vi "CODMn通讯.vi"() -> ()   [LabVIEW 2016, in "斯坦道CODMn.lvlib"]
uses:
  <vilib>/NI/Modbus Library/API/Wrapper/Create TCP Slave.vi
  <vilib>/NI/Modbus Library/API/slave/Modbus Slave.lvclass
  <vilib>/Plasmionique/MB Master/MB_Master/MB_Master.lvclass
  <vilib>/Plasmionique/MB Master/MB Master.lvlib
  <vilib>/Utility/config.llb/NI_LVConfig.lvlib
  <vilib>/NI/Modbus Library/API/Wrapper/API Main.lvlib
panel:
  in  "读取数据":bool
  in  "释放串口":bool
  in  "打开串口":bool
  out "队列中元素数量":i32
  out "元素":cluster{"命令":string}[](array[cluster])
  out "待处理插入数量":i32
  out "读取公式":u16[](array[numeric])
  out "读取参数":u16[](array[numeric])
  out "数据存储":u16[](array[numeric])
  out "温度":bool[](array[boolean])
  out "M输出点":bool[](array[boolean])
  out "ORP、时间":u16[](array[numeric])
  out "测量状态":u16[](array[numeric])
  out "通讯状态":bool
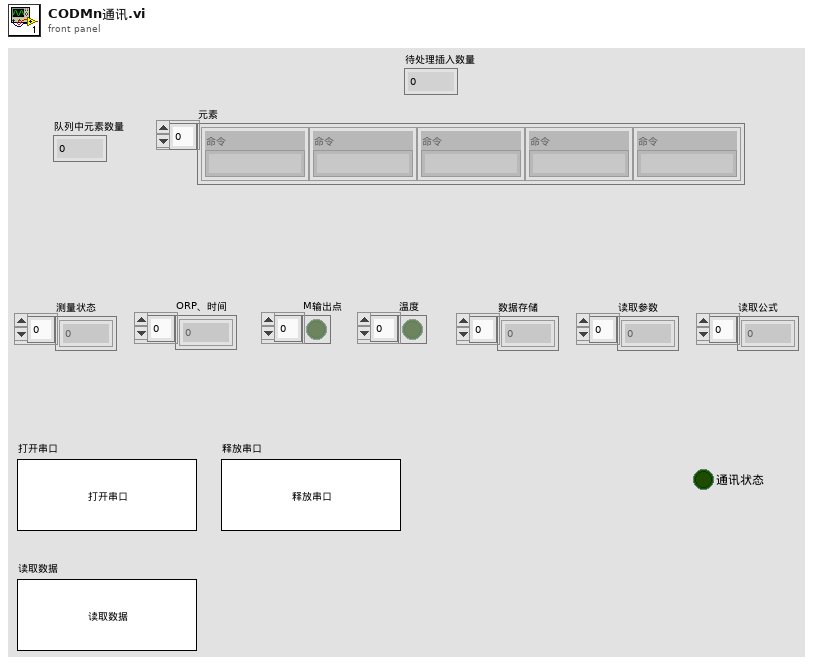
[diagram p1: front panel]
types:
  T1 = typedef "NI_LVConfig.lvlib/Config Data RefNum.ctl" = refnum<k1>
  T2 = enum16{"空闲", "水样测试", "标样核查", "零点核查", "跨度核查", "空白测试", "平行样测试", "质控样", "空白校准", "标样校准", "加标回收"}
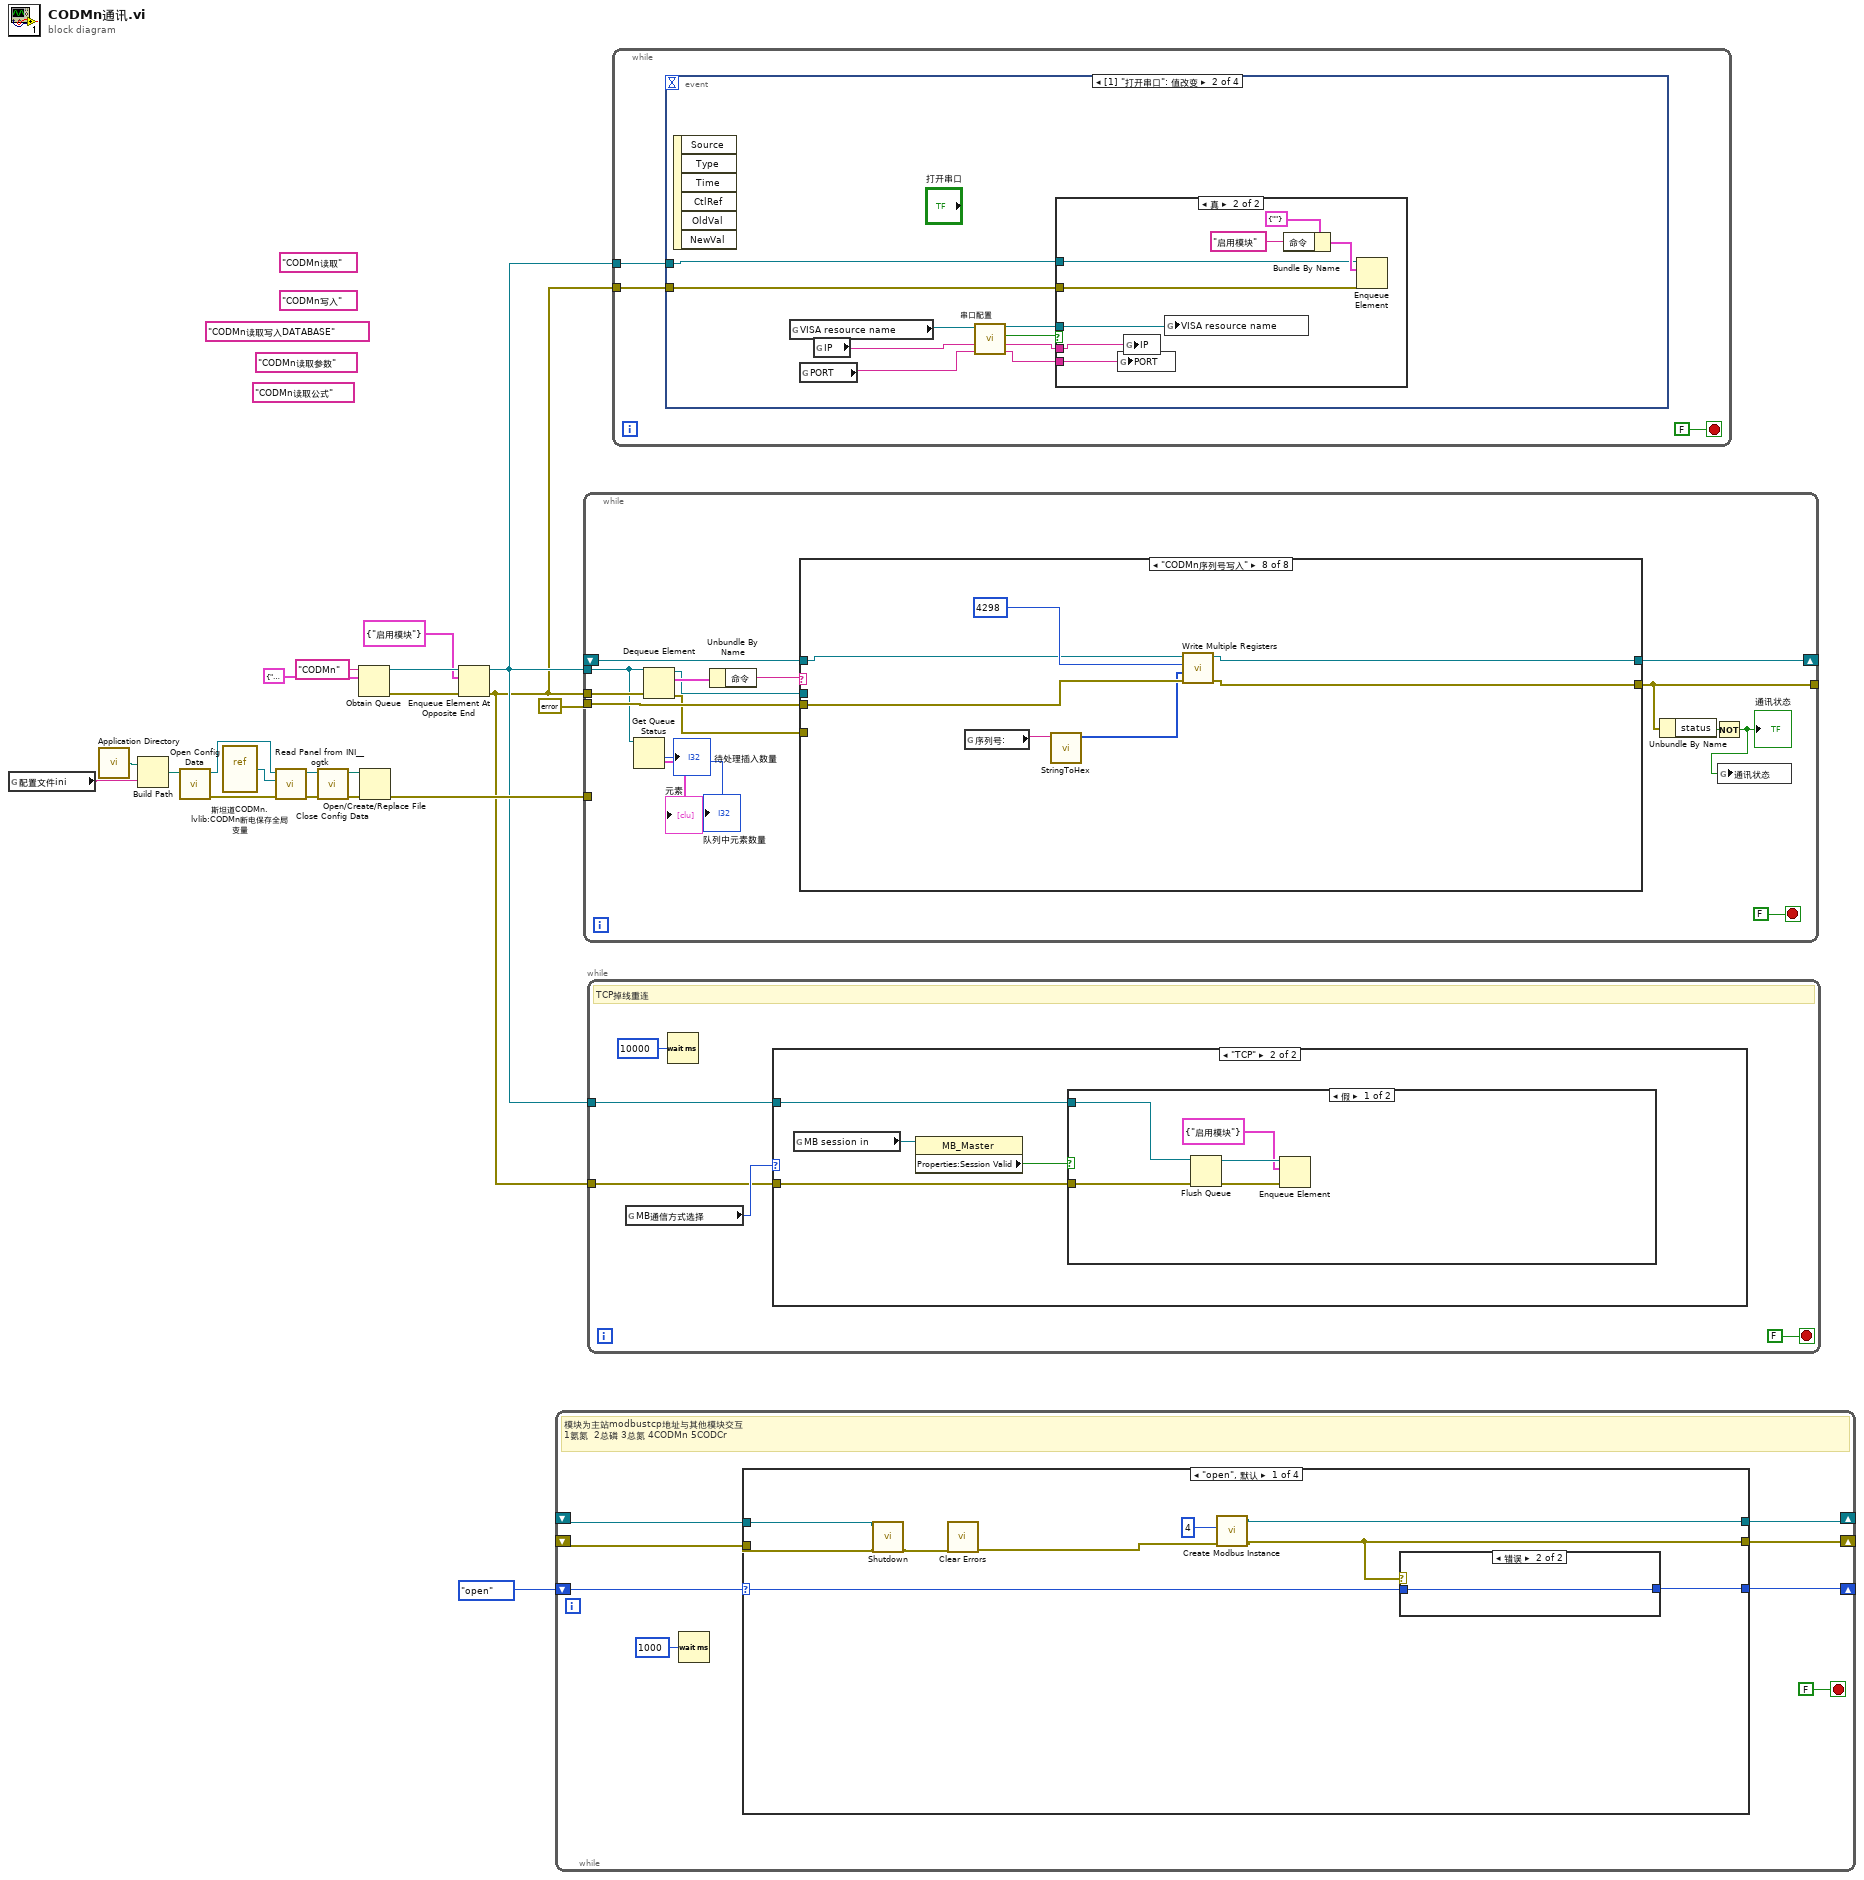
[diagram p0: block diagram]
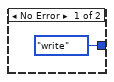
[diagram p4: hidden frame]
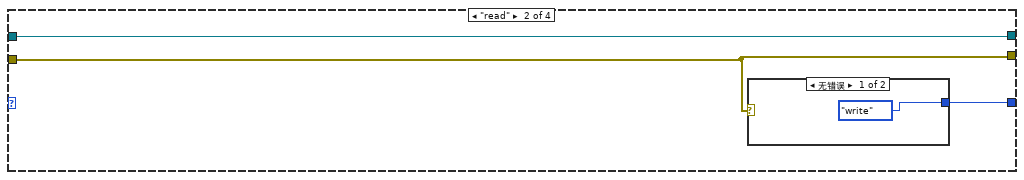
[diagram p5: hidden frame]
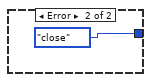
[diagram p6: hidden frame]
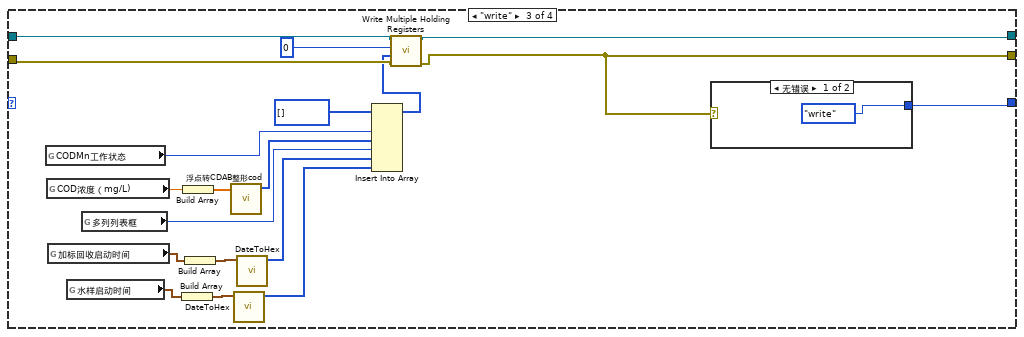
[diagram p7: hidden frame]
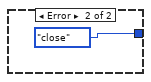
[diagram p8: hidden frame]
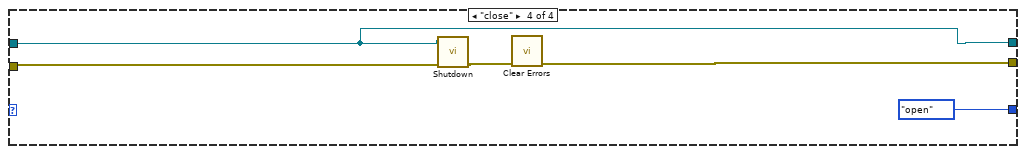
[diagram p9: hidden frame]
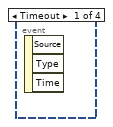
[diagram p10: hidden frame]
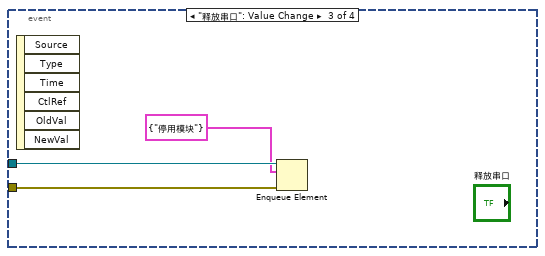
[diagram p12: hidden frame]
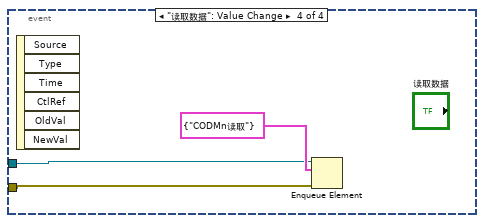
[diagram p13: hidden frame]
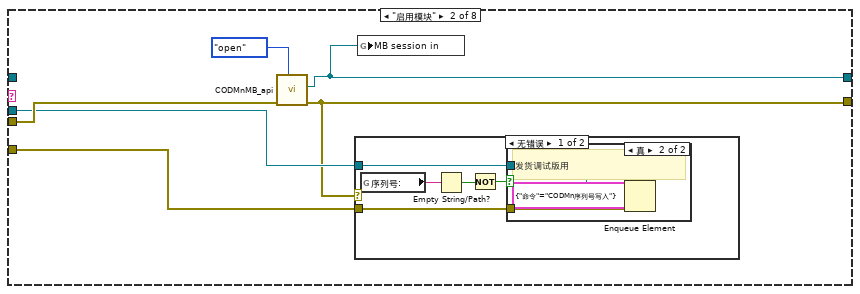
[diagram p15: hidden frame]
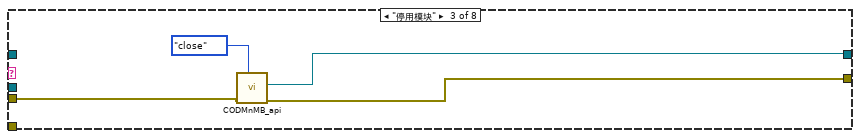
[diagram p18: hidden frame]
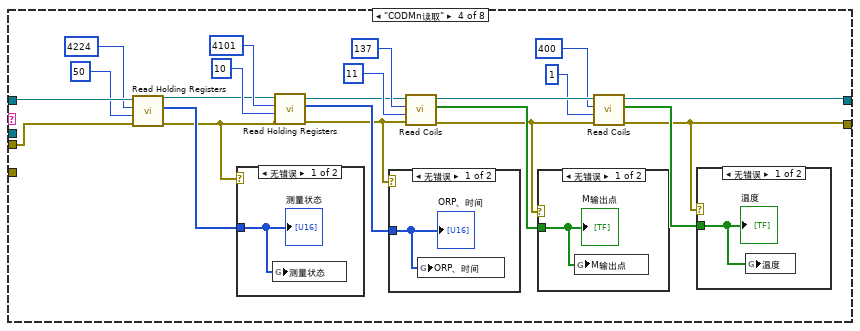
[diagram p19: hidden frame]
diagram:
  (unwired) "CODMn读取公式" ("名称（未命名）")
  (unwired) "CODMn读取写入DATABASE" ("名称（未命名）")
  (unwired) "CODMn读取参数" ("名称（未命名）")
  (unwired) "CODMn读取" ("名称（未命名）")
  (unwired) "CODMn写入" ("名称（未命名）")
  n1 = global read "COD读取DATA全局.vi" "配置文件ini"() -> (w1:string)
  n2 = call <vilib>:"Application Directory.vi"() -> ("Application Directory"=w14:path)
  n3 = Build Path(base path=w14, name or relative path=w1) -> (appended path=w13:path)
  n4 = call <vilib>:"Open Config Data.vi"("configuration file path"=w13) -> ("error out"=w9:errorcluster, "refnum"=w12:T1)  [unwired: 8 in, 1 out]
  n5 = vi-ref "斯坦道CODMn.lvlib:CODMn断电保存全局变量.vi"() -> (w11:refnum<vi>)
  n6 = call <userlib>:"Read Panel from INI__ogtk.vi"("error in (no error)"=w9, "VI ref"=w11, "refnum"=w12) -> ("error out"=w8:errorcluster, "refnum out"=w10:T1)  [unwired: 7 in]
  n7 = call <vilib>:"Close Config Data.vi"("error in (no error)"=w8, "refnum"=w10) -> ("error out"=w7:errorcluster, "file path"=w6:path)  [unwired: 8 in]
  n8 = Obtain Queue(name (unnamed)="CODMn" ("名称（未命名）"), element data type=cluster{"命令":string} {"命令"="启用模块"} ("元素")) -> (queue out=w17:refnum<queue>, error out=w16:errorcluster)  [unwired: 3 in, 1 out]
  n9 = Open/Create/Replace File(file path (use dialog)=w6, error in=w7) -> (error out=w5:errorcluster)  [unwired: 4 in, 2 out]
  n10 = Enqueue Element At Opposite End(queue=w17, element=cluster{"命令":string} {"命令"="启用模块"} ("元素"), error in (no error)=w16) -> (queue out=w3:refnum<queue>, error out=w2:errorcluster)  [unwired: 1 in, 1 out]
  n11 = while {
    shift-right: [w26] -> _
    shift-left: _ -> [w28]
    shift-right: [w25] -> _
    shift-left: _ -> [w27]
    shift-right: [w22] -> _
    shift-left: enum16{"open", "read", "write", "close"}."open" -> [w23]
    stop <- FALSE stop-if-true
    # "模块为主站modbustcp地址与其他模块交互\n1氨氮  2总磷 3总氮 4CODMn 5CODCr"
    n12 = Wait (ms)(milliseconds to wait=u32 1000 ("等待时间（毫秒）")) -> ()  [unwired: 1 out]
    n13 = case shown="\"open\", 默认" w23 {
      selector: w23 -> [w37 _ _ _]
      tunnel: w28 -> [w31 w40 w62 w68]
      tunnel: w27 -> [w30 w41 w59 w67]
      tunnel: [w34 w40 w61 w68] -> w26
      tunnel: [w33 w41 w60 w70] -> w25
      tunnel: [w36 w42 w63 enum16{"open", "read", "write", "close"}."open"] -> w22
      frame "open", Default {
        n14 = call-dynamic "Shutdown.vi"("error in"=w30, "Modbus slave in"=w31) -> ("error out"=w29:errorcluster)  [unwired: 9 in]
        n15 = call <vilib>:"Clear Errors.vi"("error in (no error)"=w29) -> ("error out"=w32:errorcluster)  [unwired: 5 in, 1 out]
        n16 = call-poly <vilib>:"Create Modbus Instance.vi"("error in"=w32, "port (502)"=u16 4) -> ("error out"=w33:errorcluster, "TCP slave instance"=w34:refnum<class "Modbus Slave.lvclass">)  [unwired: 8 in]
        n17 = case shown="错误" w33 {
          tunnel: w37 -> [_ w39]
          tunnel: [enum16{"open", "read", "write", "close"}."write" w39] -> w36
          frame No Error {
          }
          frame Error {
          }
        }
      }
      frame "read" {
        n18 = case shown="无错误" w41 {
          tunnel: [enum16{"open", "read", "write", "close"}."write" enum16{"open", "read", "write", "close"}."close"] -> w42
          frame No Error {
          }
          frame Error {
          }
        }
      }
      frame "write" {
        n19 = global read "COD测量模式全局.vi" "CODMn工作状态"() -> (w49:T2)
        n20 = global read "COD浓度全局变量.vi" "COD浓度（mg/L)"() -> (w51:dbl)
        n21 = global read "COD测量模式全局.vi" "加标回收启动时间"() -> (w54:timestamp)
        n22 = global read "COD测量模式全局.vi" "水样启动时间"() -> (w56:timestamp)
        n23 = global read "运行时序全局变量.vi" "多列列表框"() -> (w53:i32)
        n24 = Build Array(w56) -> (w55:timestamp[])
        n25 = Build Array(w51) -> (w50:dbl[])
        n26 = Build Array(w54) -> (w47:timestamp[])
        n27 = call "浮点转CDAB整形cod.vi"("浮点数"=w50) -> ("CDAB整形输出"=w52:u16[])  [unwired: 10 in]
        n28 = call "DateToHex.vi"("DATE"=w55) -> ("数组"=w58:u16[])  [unwired: 10 in]
        n29 = call "DateToHex.vi"("DATE"=w47) -> ("数组"=w57:u16[])  [unwired: 10 in]
        n30 = Insert Into Array(array=u16[] [] ("values"), new element #1=w49, new element #2=w52, new element #3=w53, new element #4=w57, new element #5=w58) -> (w46:u16[])  [unwired: 1 in]
        n31 = call-dynamic "Write Multiple Holding Registers.vi"("error in"=w59, "registers to write"=w46, "starting address"=u16 0, "Modbus slave in"=w62) -> ("error out"=w60:errorcluster, "Modbus slave out"=w61:refnum<class "Modbus Slave.lvclass">)  [unwired: 6 in]
        n32 = case shown="无错误" w60 {
          tunnel: [enum16{"open", "read", "write", "close"}."write" enum16{"open", "read", "write", "close"}."close"] -> w63
          frame No Error {
          }
          frame Error {
          }
        }
      }
      frame "close" {
        n33 = call-dynamic "Shutdown.vi"("error in"=w67, "Modbus slave in"=w68) -> ("error out"=w66:errorcluster)  [unwired: 9 in]
        n34 = call <vilib>:"Clear Errors.vi"("error in (no error)"=w66) -> ("error out"=w70:errorcluster)  [unwired: 5 in, 1 out]
      }
    }
  }
  n35 = while {
    tunnel: w3 -> [w76]
    tunnel: w2 -> [w85]
    tunnel: [w77] -> _
    shift-right: [w81] -> _
    shift-left: _ -> [w80]
    tunnel: errorcluster {"status"=FALSE, "code"=0, "source"=""} ("error out") -> [w79]
    tunnel: w5 -> [_]
    stop <- FALSE stop-if-true
    n36 = Get Queue Status(queue=w76) -> (# pending insert=→"待处理插入数量":i32, # elements in queue=→"队列中元素数量":i32, elements=→"元素":cluster{"命令":string}[])  [unwired: 2 in, 5 out]
    n37 = Dequeue Element(queue=w76, error in (no error)=w85) -> (queue out=w72:refnum<queue>, element=w84:cluster{"命令":string}, error out=w71:errorcluster)  [unwired: 1 in, 1 out]
    n38 = Unbundle By Name(w84) -> ("命令"=w83:string)
    n39 = case shown="\"CODMn序列号写入\"" w83 {
      tunnel: [w88 w92 w103 w114 w135 w144 w161 w168] -> w81
      tunnel: [w87 w89 w104 w107 w133 w143 w160 w167] -> w77
      tunnel: w80 -> [w88 _ _ w128 w139 w153 w164 w172]
      tunnel: w79 -> [w87 w93 w105 w127 w136 w152 w163 w171]
      tunnel: w72 -> [_ w91 _ _ _ _ _ _]
      tunnel: w71 -> [_ w90 _ _ _ _ _ _]
      frame Default {
      }
      frame "启用模块" {
        n40 = call "CODMnMB_api.vi"("STEP"=enum16{"open", "read", "write", "close"}."open", "Error in"=w93) -> ("error out"=w89:errorcluster, "MB session out"=w92:refnum<class "MB_Master.lvclass">)  [unwired: 7 in, 1 out]
        n41 = case shown="无错误" w89 {
          tunnel: w91 -> [w99 _]
          tunnel: w90 -> [w96 _]
          frame No Error {
            n42 = global read "COD读取DATA全局.vi" "序列号:"() -> (w98:string)
            n43 = Empty String/Path?(string/path=w98) -> (empty?=w97:bool)
            n44 = Not(x=w97) -> (.not. x?=w95:bool)
            n45 = case shown="真" w95 {
              tunnel: w99 -> [_ w102]
              tunnel: w96 -> [_ w101]
              frame False {
              }
              frame True {
                # "发货调试版用"
                n46 = Enqueue Element(queue=w102, element=cluster{"命令":string} {"命令"="CODMn序列号写入"} ("元素"), error in (no error)=w101) -> ()  [unwired: 1 in, 3 out]
              }
            }
          }
          frame Error {
          }
        }
        n47 = global write "COD浓度全局变量.vi" "MB session in"(w92) -> ()
      }
      frame "停用模块" {
        n48 = call "CODMnMB_api.vi"("STEP"=enum16{"open", "read", "write", "close"}."close", "Error in"=w105) -> ("error out"=w104:errorcluster, "MB session out"=w103:refnum<class "MB_Master.lvclass">)  [unwired: 7 in, 1 out]
      }
      frame "CODMn读取" {
        n49 = call <vilib>:"Read Holding Registers.vi"("error in (no error)"=w127, "quantity"=u16 50 ("number of holding registers"), "starting address"=u16 4224, "MB session in"=w128) -> ("error out"=w118:errorcluster, "Registers"=w124:u16[], "MB session out"=w119:refnum<class "MB_Master.lvclass">)  [unwired: 5 in]
        n50 = case shown="无错误" w118 {
          tunnel: w124 -> [w132 _]
          frame No Error {
            n51 = global write "COD读取DATA全局.vi" "测量状态"(w132) -> ()
            "测量状态" <- w132
          }
          frame Error {
          }
        }
        n52 = call <vilib>:"Read Holding Registers.vi"("error in (no error)"=w118, "quantity"=u16 10, "starting address"=u16 4101, "MB session in"=w119) -> ("error out"=w113:errorcluster, "Registers"=w117:u16[], "MB session out"=w116:refnum<class "MB_Master.lvclass">)  [unwired: 5 in]
        n53 = case shown="无错误" w113 {
          tunnel: w117 -> [w131 _]
          frame No Error {
            n54 = global write "COD读取DATA全局.vi" "ORP、时间"(w131) -> ()
            "ORP、时间" <- w131
          }
          frame Error {
          }
        }
        n55 = call <vilib>:"Read Coils.vi"("error in (no error)"=w113, "quantity"=u16 11, "starting address"=u16 137, "MB session in"=w116) -> ("error out"=w111:errorcluster, "Coils"=w112:bool[], "MB session out"=w115:refnum<class "MB_Master.lvclass">)  [unwired: 5 in]
        n56 = case shown="无错误" w111 {
          tunnel: w112 -> [w130 _]
          frame No Error {
            n57 = global write "COD读取DATA全局.vi" "M输出点"(w130) -> ()
            "M输出点" <- w130
          }
          frame Error {
          }
        }
        n58 = call <vilib>:"Read Coils.vi"("error in (no error)"=w111, "quantity"=u16 1, "starting address"=u16 400, "MB session in"=w115) -> ("error out"=w107:errorcluster, "Coils"=w108:bool[], "MB session out"=w114:refnum<class "MB_Master.lvclass">)  [unwired: 5 in]
        n59 = case shown="无错误" w107 {
          tunnel: w108 -> [w129 _]
          frame No Error {
            n60 = global write "COD读取DATA全局.vi" "温度"(w129) -> ()
            "温度" <- w129
          }
          frame Error {
          }
        }
      }
      frame "CODMn读取写入DATABASE" {
        n61 = call <vilib>:"Read Holding Registers.vi"("error in (no error)"=w136, "quantity"=u16 10 ("number of holding registers"), "starting address"=u16 4101, "MB session in"=w139) -> ("error out"=w133:errorcluster, "Registers"=w134:u16[], "MB session out"=w135:refnum<class "MB_Master.lvclass">)  [unwired: 5 in]
        n62 = case shown="无错误" w133 {
          tunnel: w134 -> [w141 _]
          frame No Error {
            n63 = global write "COD读取DATA全局.vi" "数据存储"(w141) -> ()
            n64 = global write "COD读取DATA全局.vi" "读取写入data"(TRUE ("读取参数显示")) -> ()
            "数据存储" <- w141
          }
          frame Error {
          }
        }
      }
      frame "CODMn读取参数" {
        n65 = call <vilib>:"Read Holding Registers.vi"("error in (no error)"=w152, "quantity"=u16 35 ("number of holding registers"), "starting address"=u16 4272, "MB session in"=w153) -> ("error out"=w147:errorcluster, "Registers"=w149:u16[], "MB session out"=w148:refnum<class "MB_Master.lvclass">)  [unwired: 5 in]
        n66 = case shown="无错误" w147 {
          tunnel: w149 -> [w157 _]
          frame No Error {
            n67 = global write "COD读取DATA全局.vi" "读取参数"(w157) -> ()
            n68 = global write "COD读取DATA全局.vi" "读取参数显示"(TRUE ("读取参数显示")) -> ()
            "读取参数" <- w157
          }
          frame Error {
          }
        }
        n69 = call <vilib>:"Read Holding Registers.vi"("error in (no error)"=w147, "quantity"=u16 4, "starting address"=u16 5596, "MB session in"=w148) -> ("error out"=w143:errorcluster, "Registers"=w142:u16[], "MB session out"=w144:refnum<class "MB_Master.lvclass">)  [unwired: 5 in]
        n70 = case shown="无错误" w143 {
          tunnel: w142 -> [w155 _]
          frame No Error {
            n71 = global write "COD读取DATA全局.vi" "读取浮台参数"(w155) -> ()
            n72 = global write "COD读取DATA全局.vi" "读取浮台参数显示"(TRUE ("读取参数显示")) -> ()
          }
          frame Error {
          }
        }
      }
      frame "CODMn读取公式" {
        n73 = call <vilib>:"Read Holding Registers.vi"("error in (no error)"=w163, "quantity"=u16 94 ("number of holding registers"), "starting address"=u16 4616, "MB session in"=w164) -> ("error out"=w160:errorcluster, "Registers"=w162:u16[], "MB session out"=w161:refnum<class "MB_Master.lvclass">)  [unwired: 5 in]
        n74 = case shown="无错误" w160 {
          tunnel: w162 -> [w166 _]
          frame No Error {
            n75 = global write "COD读取DATA全局.vi" "读取公式"(w166) -> ()
            n76 = global write "COD读取DATA全局.vi" "读取公式显示"(TRUE ("读取参数显示")) -> ()
            "读取公式" <- w166
          }
          frame Error {
          }
        }
      }
      frame "CODMn序列号写入" {
        n77 = global read "COD读取DATA全局.vi" "序列号:"() -> (w170:string)
        n78 = call "StringToHex.vi"("STRING"=w170) -> ("数组"=w169:u16[])  [unwired: 10 in]
        n79 = call <vilib>:"Write Multiple Registers.vi"("error in (no error)"=w171, "values"=w169, "starting address"=u16 4298, "MB session in"=w172) -> ("error out"=w167:errorcluster, "MB session out"=w168:refnum<class "MB_Master.lvclass">)  [unwired: 6 in]
      }
    }
    n80 = Unbundle By Name(w77) -> ("status"=w82:bool)
    n81 = Not(x=w82) -> (.not. x?=w78:bool)
    "通讯状态" <- w78
    n82 = global write "COD读取DATA全局.vi" "通讯状态"(w78) -> ()
  }
  n83 = while "While循环" {
    tunnel: w3 -> [w175]
    tunnel: w2 -> [w174]
    stop <- FALSE stop-if-true
    # "TCP掉线重连"
    n84 = global read "CODMn断电保存全局变量.vi" "MB通信方式选择"() -> (w176:enum16{"串口", "TCP"})
    n85 = Wait (ms)(milliseconds to wait=u32 10000 ("等待时间（毫秒）")) -> ()  [unwired: 1 out]
    n86 = case shown="\"TCP\"" w176 {
      tunnel: w175 -> [_ w180]
      tunnel: w174 -> [_ w179]
      frame "串口", Default {
      }
      frame "TCP" {
        n87 = global read "COD浓度全局变量.vi" "MB session in"() -> (w182:refnum<class "MB_Master.lvclass">)
        n88 = property class="MB_Master"(reference=w182) -> ("Properties:Session Valid"=w181:bool)  [unwired: 1 in, 2 out]
        n89 = case shown="假" w181 {
          tunnel: w180 -> [w184 _]
          tunnel: w179 -> [w183 _]
          frame False {
            n90 = Flush Queue(queue=w184, error in (no error)=w183) -> (queue out=w187:refnum<queue>, error out=w186:errorcluster)  [unwired: 1 out]
            n91 = Enqueue Element(queue=w187, element=cluster{"命令":string} {"命令"="启用模块"} ("元素"), error in (no error)=w186) -> ()  [unwired: 1 in, 3 out]
          }
          frame True {
          }
        }
      }
    }
  }
  n92 = while {
    tunnel: w3 -> [w189]
    tunnel: w2 -> [w188]
    stop <- FALSE stop-if-true
    n93 = event shown="[1] \"打开串口\": 值改变" {
      selector: _ -> [_ _ _ _]
      dyn-events: _ -> [_ _ _ _]
      timeout: _ -> [_ _ _ _]
      tunnel: w189 -> [_ w196 w210 w212]
      tunnel: w188 -> [_ w195 w209 w211]
      event Timeout {
        n94 = event-data() -> ()  [unwired: 1 in, 3 out]
      }
      event "打开串口": Value Change {
        n95 = event-data() -> ()  [unwired: 1 in, 6 out]
        n96 = global read "CODMn断电保存全局变量.vi" "VISA resource name"() -> (w199:refnum<visa-resource-name>)
        n97 = global read "CODMn断电保存全局变量.vi" "PORT"() -> (w191:string)
        n98 = global read "CODMn断电保存全局变量.vi" "IP"() -> (w192:string)
        n99 = call "串口配置.vi"("PORT"=w191, "IP"=w192, "请选择串口:"=w199) -> ("PORT 2"=w193:string, "IP 2"=w194:string, "确认 2"=w197:bool, "VISA资源名称 2"=w198:refnum<visa-resource-name>)  [unwired: 4 in, 1 out]
        n100 = case shown="真" w197 {
          tunnel: w198 -> [_ w207]
          tunnel: w196 -> [_ w203]
          tunnel: w195 -> [_ w202]
          tunnel: w194 -> [_ w201]
          tunnel: w193 -> [_ w200]
          frame False {
          }
          frame True {
            n101 = global write "CODMn断电保存全局变量.vi" "PORT"(w200) -> ()
            n102 = global write "CODMn断电保存全局变量.vi" "IP"(w201) -> ()
            n103 = global write "CODMn断电保存全局变量.vi" "VISA resource name"(w207) -> ()
            n104 = Bundle By Name(cluster=cluster{"命令":string} {"命令"=""} ("元素"), "命令"="启用模块" ("名称（未命名）")) -> (w204:cluster{"命令":string})
            n105 = Enqueue Element(queue=w203, element=w204, error in (no error)=w202) -> ()  [unwired: 1 in, 3 out]
          }
        }
      }
      event "释放串口": Value Change {
        n106 = event-data() -> ()  [unwired: 1 in, 6 out]
        n107 = Enqueue Element(queue=w210, element=cluster{"命令":string} {"命令"="停用模块"} ("元素"), error in (no error)=w209) -> ()  [unwired: 1 in, 3 out]
      }
      event "读取数据": Value Change {
        n108 = event-data() -> ()  [unwired: 1 in, 6 out]
        n109 = Enqueue Element(queue=w212, element=cluster{"命令":string} {"命令"="CODMn读取"} ("元素"), error in (no error)=w211) -> ()  [unwired: 1 in, 3 out]
      }
    }
  }
